vi "Get Cell Pressures and Temperatures.vi"(0 "EUs":dbl[](array[numeric]) format="%.1f", 1 "Cell #":i32, 2 "Cell x Data":T1 {"Rw Temp" format="%.2f"; "Rw" format="%.2f"; "DAQ Units" items=["Mins", "Hrs"]; "CurData" format="%.3f"; "Last Pore Vol" format="%.3f"; "Amplitude" format="%.3f"; "ElectSpace" format="%.2f"; "Permeability" format="%.2f"; "Porosity" format="%.2f"; "Diameter" format="%.2f"; "Length" format="%.2f"}, 3 "No Galil":bool[](array[boolean])) -> (14 "T-A":dbl format="%.2f", 15 "T-B":dbl format="%.2f", 16 "NOP":dbl format="%.2f", 17 "Pc":dbl format="%.2f", 18 "Delta-P":dbl format="%.2f", 19 "DwnStrm-P":dbl format="%.2f")   [LabVIEW 2013]
panel:
  in  "Cell-to-EU Index Matrix":i32[][](array[numeric])=[[1, 8, 12, 22, 26], [2, 9, 13, 23, 27], [0, 7, 17, 21, 31], [4, 14, 11, 28, 25], [3, 10, 18, 24, 32], [35, 37, 39, 41, 43], [0, 0, 0, 0, 0]]
  # "T-A\n\nT-B\n\nNOP\n\nPc-Lo\n\nPc-Hi\n\nDelta-P\n\nDnstrm P"
  # "Cell-1   Cell-2   Cell-3   Cell-4    Cell-5"
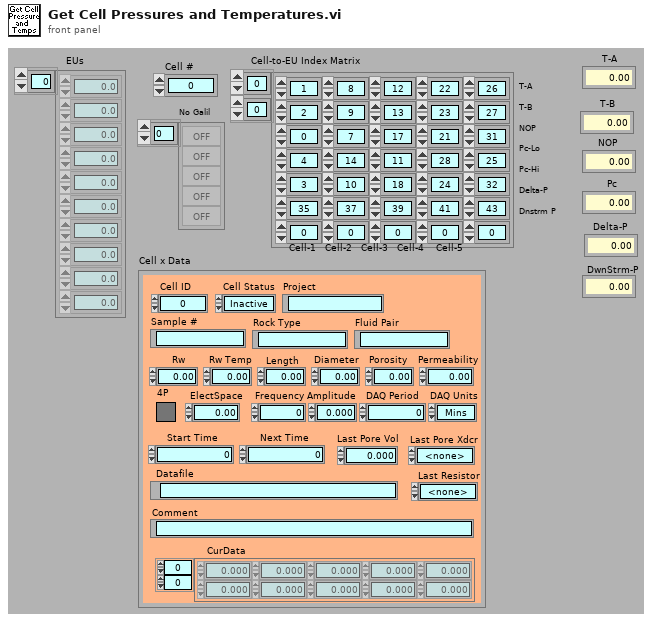
[diagram p1: front panel]
types:
  T1 = cluster{"Cell ID":i32, "Cell Status":enum16{"Inactive", "Setup", "Active", "Done"}, "Project":string, "Sample #":string, "Rock Type":string, "Fluid Pair":string, "Rw":dbl, "Rw Temp":dbl, "Length":dbl, "Diameter":dbl, "Porosity":dbl, "Permeability":dbl, "4P":bool, "ElectSpace":dbl, "Frequency":dbl, "Amplitude":dbl, "DAQ Period":u32, "DAQ Units":u16, "Start Time":dbl, "Next Time":dbl, "Datafile":path, "Last Pore Vol":dbl, "Last Pore Xdcr":enum16{"<none>", "Lo Range", "Hi Range"}, "Last Resistor":enum16{"<none>", "Resistor 1", "Resistor 2", "Resistor 3", "Resistor 4", "Resistor 5", "Resistor 6"}, "CurData":dbl[][], "Comment":string}
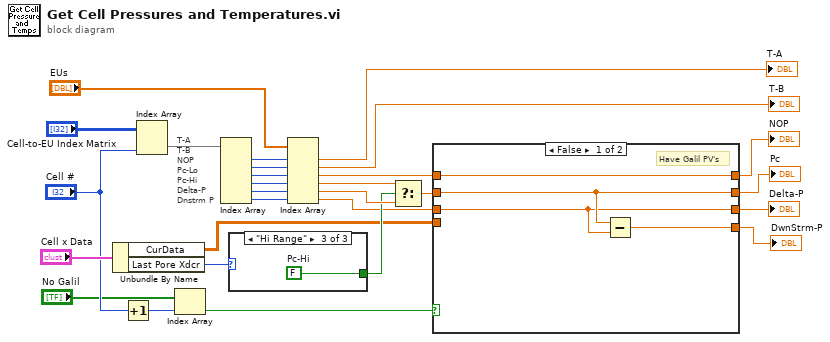
[diagram p0: block diagram]
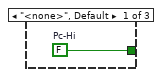
[diagram p2: hidden frame]
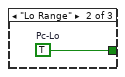
[diagram p3: hidden frame]
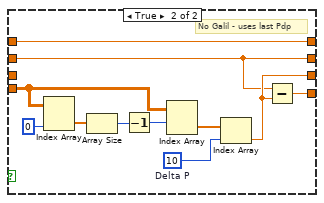
[diagram p4: hidden frame]
diagram:
  # "T-A\nT-B\nNOP\nPc-Lo\nPc-Hi\nDelta-P\nDnstrm P"
  n1 = Unbundle By Name("Cell x Data") -> ("CurData"=w2:dbl[][], "Last Pore Xdcr"=w11:enum16{"<none>", "Lo Range", "Hi Range"})
  n2 = Increment(x="Cell #") -> (x+1=w15:i32)
  n3 = Index Array(array="Cell-to-EU Index Matrix", index (col)="Cell #") -> (element=w26:i32[])  [unwired: 1 in]
  n4 = Index Array(array="No Galil", index=w15) -> (element=w1:bool)
  n5 = Index Array(array=w26) -> (element #1=w25:i32, element #2=w24:i32, element #3=w23:i32, element #4=w22:i32, element #5=w21:i32, element #6=w20:i32)  [unwired: 6 in]
  n6 = case shown="\"Hi Range\"" w11 {
    tunnel: [w29 w30 w31] -> w10
    frame "<none>", Default {
      w29 = FALSE  # Pc-Hi
    }
    frame "Lo Range" {
      w30 = TRUE  # Pc-Lo
    }
    frame "Hi Range" {
      w31 = FALSE  # Pc-Hi
    }
  }
  n7 = Index Array(array="EUs", index #1=w25, index #2=w24, index #3=w23, index #4=w22, index #5=w21, index #6=w20) -> (element #1=→"T-A":dbl, element #2=→"T-B":dbl, element #3=w9:dbl, element #4=w13:dbl, element #5=w12:dbl, element #6=w7:dbl)
  n8 = Select(t=w13, s=w10, f=w12) -> (s? t:f=w8:dbl)
  n9 = case shown="False" w1 {
    tunnel: [w34 w38] -> w6
    tunnel: [w33 w37] -> w5
    tunnel: [w32 w39] -> w4
    tunnel: [w35 w40] -> w3
    tunnel: w9 -> [w34 w38]
    tunnel: w8 -> [w33 w37]
    tunnel: w7 -> [w32 _]
    tunnel: w2 -> [_ w36]
    frame False {
      # "Have Galil PV's"
      n10 = Subtract(x=w33, y=w32) -> (x-y=w35:dbl)
    }
    frame True {
      w42 = 10  # Delta P
      # "No Galil - uses last Pdp"
      n11 = Index Array(array=w36, index (col)=0 ("disabled index (col)")) -> (element=w45:dbl[])  [unwired: 1 in]
      n12 = Array Size(array=w45) -> (size(s)=w44:i32)
      n13 = Decrement(x=w44) -> (x-1=w41:i32)
      n14 = Index Array(array=w36, index (row)=w41) -> (element=w43:dbl[])  [unwired: 1 in]
      n15 = Index Array(array=w43, index=w42) -> (element=w39:dbl)
      n16 = Subtract(x=w37, y=w39) -> (x-y=w40:dbl)
    }
  }
  "NOP" <- w6
  "Pc" <- w5
  "Delta-P" <- w4
  "DwnStrm-P" <- w3
